vi "Find Visa Recorders.vi"(8 "Error In":errorcluster, 10 "Timeout":i32=500) -> (0 "Error Out":errorcluster, 2 "Names":string[](array[string]), 3 "Recorders List":refnum<class "Instrument Actor.lvclass">[](array[class]))   [LabVIEW 2020]
uses:
  Instrument Actor/Instrument Actor.lvclass
  <vilib>/Instr/_visa.llb/VISA Find Search Mode.ctl
panel:
  out "find list":refnum<visa-resource-name>[](array[refnum])
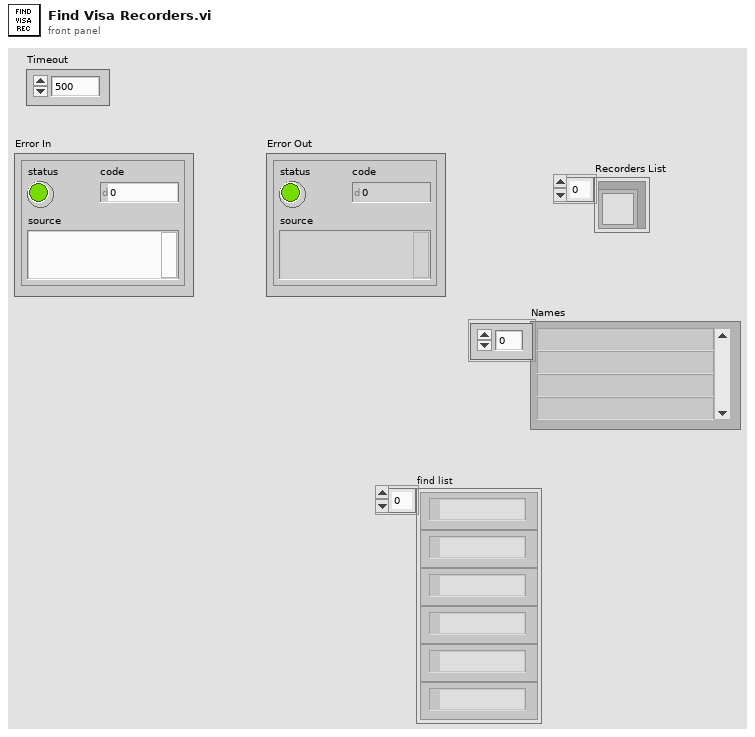
[diagram p1: front panel]
types:
  T1 = typedef "VISA Find Search Mode.ctl" = u32
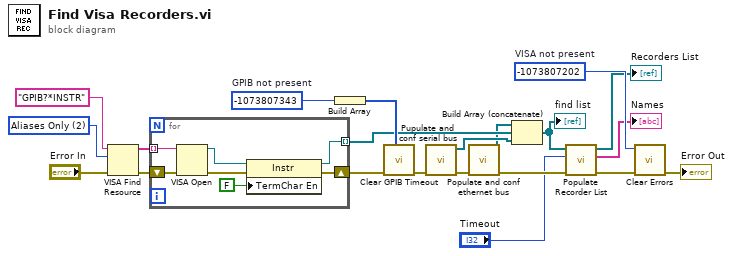
[diagram p0: block diagram]
diagram:
  w11 = -1073807202  # VISA not present
  w18 = -1073807343  # GPIB not present
  w20 = T1 2 items=["Canonical Names Only"=0, "Aliases Only"=2, "Include Matching Aliases"=3, "Include All Aliases"=4] ("Search Mode")
  n1 = VISA Find Resource(8:"Error In", 10:w20, 11:"GPIB?*INSTR" ("expression (\"?*\")")) -> (0:w15:errorcluster, 3:w13:string[])  [unwired: 1 out]
  n2 = for {
    shift-right: [w24] -> w14
    shift-left: w15 -> [w26]
    tunnel: w13 -> [w28] mode=indexing
    tunnel: [w23] -> w12 mode=indexing
    n3 = VISA Open(error in (no error)=w26, VISA resource name=w28) -> (VISA resource name=w27:refnum<visa-resource-name>, error out=w25:errorcluster)  [unwired: 3 in]
    n4 = property class="Instr"(reference=w27, error in=w25, "TermChar En"=FALSE ("Message Based Settings:Termination Character Enable")) -> (reference out=w23:refnum<visa-resource-name>, error out=w24:errorcluster)
  }
  n5 = Build Array(w18) -> (w17:i32[])
  n6 = call "Clear GPIB Timeout.vi"("Errors to skip"=w17, "error in (no error)"=w14) -> ("error out"=w16:errorcluster)  [unwired: 9 out]
  n7 = call "Pupulate and conf serial bus.vi"("Error In"=w16) -> ("Error Out"=w4:errorcluster, "Devices"=w19:refnum<visa-resource-name>[])  [unwired: 9 in]
  n8 = call "Populate and conf ethernet bus.vi"("Error In"=w4) -> ("Error Out"=w3:errorcluster, "Devices"=w2:refnum<visa-resource-name>[])  [unwired: 9 in]
  n9 = Build Array (concatenate)(w2, w12, w19) -> (w8:refnum<visa-resource-name>[])
  "find list" <- w8
  n10 = call "Populate Recorder List.vi"("error in (no error)"=w3, "Timeout"="Timeout", "VISA Resourse Names"=w8) -> ("error out"=w7:errorcluster, "Names"=→"Names":string[], "Instrument List"=→"Recorders List":refnum<class "Instrument Actor.lvclass">[])  [unwired: 6 in]
  n11 = call <vilib>:"Clear Errors.vi"("error in (no error)"=w7, "specific error code to clear (0: all)"=w11) -> ("error out"=→"Error Out":errorcluster)  [unwired: 4 in, 1 out]
